vi "Multi_FTP_Put2.vi"(0 "Address":string, 1 "User":string, 3 "Password":string, 5 "trj file path 2":path[](array[path]), 9 "XPS error in(no error)":errorcluster, 11 "error in (no error)":errorcluster, 12 "Cible Directory":string) -> (10 "XPS error out":errorcluster, 15 "error out":errorcluster)   [LabVIEW 2009]
panel:
  out "concatenated string":string
  out "String":string
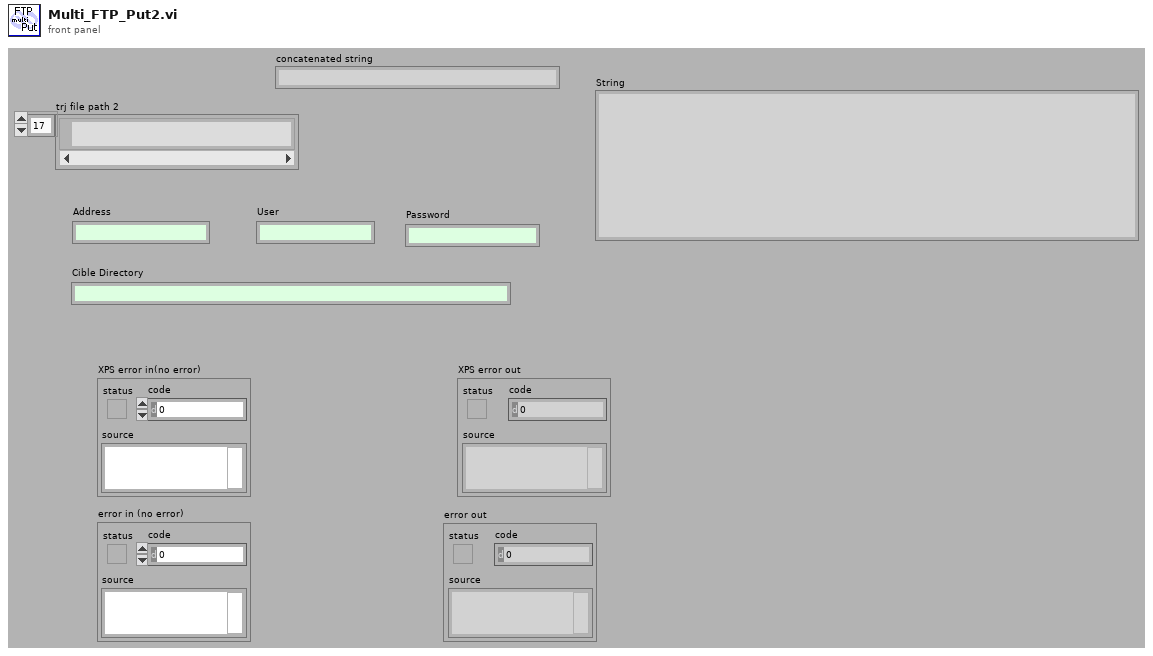
[diagram p1: front panel]
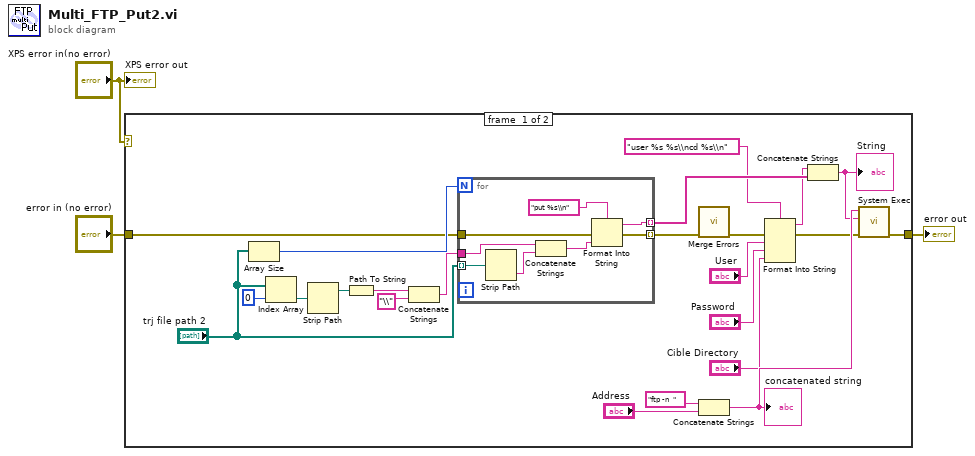
[diagram p0: block diagram]
diagram:
  n1 = case shown="No Error" "XPS error in(no error)" {
    tunnel: [w26 w35] -> w2
    tunnel: "error in (no error)" -> [w6 w35]
    frame #0 {
      n2 = Array Size(array="trj file path 2") -> (size(s)=w19:i32)
      n3 = Index Array(array="trj file path 2", index=0) -> (element=w22:path)
      n4 = Strip Path(path=w22) -> (stripped path=w21:path)  [unwired: 1 out]
      n5 = Path To String(path=w21) -> (string=w24:string)
      n6 = Concatenate Strings(w24, "\\") -> (w18:string)
      n7 = for {
        N: w19 -> [_]
        tunnel: "trj file path 2" -> [w34] mode=indexing
        tunnel: w18 -> [w33]
        tunnel: [w29] -> w17 mode=indexing
        tunnel: w6 -> [w28]
        tunnel: [w27] -> w5 mode=indexing
        n8 = Strip Path(path=w34) -> (name=w32:string)  [unwired: 1 out]
        n9 = Concatenate Strings(w33, w32) -> (w31:string)
        n10 = Format Into String(format string="put %s\\n", error in=w28, w31) -> (resulting string=w29:string, error out=w27:errorcluster)  [unwired: 1 in]
      }
      n11 = call <vilib>:"Merge Errors.vi"("error array in"=w5) -> ("error out"=w4:errorcluster)  [unwired: 6 in]
      n12 = Concatenate Strings("ftp -n  ", "Address") -> (w14:string)
      "concatenated string" <- w14
      n13 = Format Into String(format string="user %s %s\\ncd %s\\n", error in=w4, "User", "Password", "Cible Directory") -> (resulting string=w8:string, error out=w11:errorcluster)  [unwired: 1 in]
      n14 = Concatenate Strings(w8, w17) -> (w7:string)
      "String" <- w7
      n15 = call <vilib>:"System Exec.vi"("error in (no error)"=w11, "standard input"=w7, "command line"=w14) -> ("error out"=w26:errorcluster)  [unwired: 3 in, 5 out]
    }
    frame #1 {
    }
  }
  "error out" <- w2
  "XPS error out" <- "XPS error in(no error)"
